vi "Main - Machine Connectivity (FGV).vi"(7 "Action":T1=enum."Write", 8 "error In":errorcluster, 10 "Status":string[](array[string]), 11 "Device Name":string[](array[string])) -> (0 "error out":errorcluster, 2 "Status out":string[](array[string]), 3 "Device Name out":string[](array[string]))   [LabVIEW 2019]
uses:
  Controls/FGV States.ctl
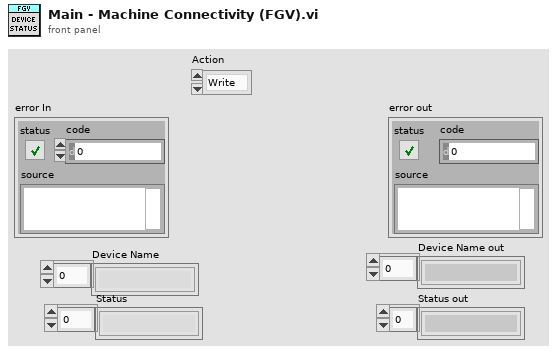
[diagram p1: front panel]
types:
  T1 = typedef "FGV States.ctl" = enum16{"Read", "Write"}
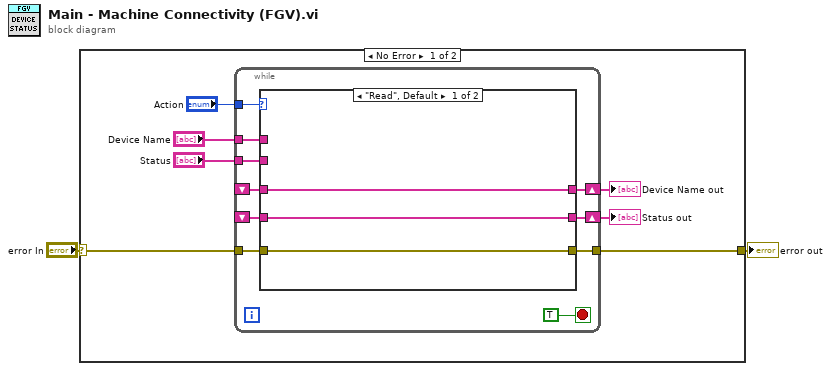
[diagram p0: block diagram]
diagram:
  n1 = case shown="No Error" "error In" {
    selector: "error In" -> [w8 w26]
    tunnel: [w7 w26] -> w1
    frame No Error {
      n2 = while {
        tunnel: "Action" -> [w19]
        tunnel: "Device Name" -> [w16]
        shift-right: [w17] -> w5
        shift-left: _ -> [w15]
        tunnel: [w14] -> w7
        tunnel: w8 -> [w13]
        tunnel: "Status" -> [w12]
        shift-right: [w11] -> w3
        shift-left: _ -> [w10]
        stop <- TRUE stop-if-true
        n3 = case shown="\"Read\", Default" w19 {
          tunnel: [w22 w25] -> w17
          tunnel: w16 -> [_ w25]
          tunnel: w15 -> [w22 _]
          tunnel: [w21 w24] -> w14
          tunnel: w13 -> [w21 w24]
          tunnel: w12 -> [_ w23]
          tunnel: [w20 w23] -> w11
          tunnel: w10 -> [w20 _]
          frame "Read", Default {
          }
          frame "Write" {
          }
        }
      }
      "Device Name out" <- w5
      "Status out" <- w3
    }
    frame Error {
    }
  }
  "error out" <- w1
